vi "Test Asic DACTH0-5.vi"(0 "Config Test IN":T1={"Config HW"={"VISA Rigol DP832"="Rigol_DP832", "Config Rigol DP832"=[{"Channel"=0, "V Limit"=5.5, "I Limit"=0.5, "V Out"=5.0}, {"Channel"=1, "V Limit"=5.5, "I Limit"=0.8, "V Out"=5.0}, {"Channel"=2, "V Limit"=5.5, "I Limit"=0.2, "V Out"=0.0}], "CTA Test#"="CTA013 A", "FT_Handle"=0, "Espera acceso FT"=10}, "Config Test"=[{"Vasic"=3.3, "Test Register?"=TRUE, "Test ADC?"=TRUE, "Test ADC"={"Repeats ADC"=100, "Max Desviation"=0.1}, "Test Max PN Min NP?"=TRUE, "Pattern Max PN Min NP"={"Max P inferior"=1.888, "Max P superior"=2.177000045776367, "Min N superior"=0.818, "Min N inferior"=0.73, "Max N superior"=1.475, "Max N inferior"=1.322, "Min P inferior "=1.321, "Min P superior"=1.474}, "Test Rate Scan?"=TRUE, "Vin Rate Scan"=[0, 1, 2, 3, 4, 5, 6, 7, 8, 9], "Test Rate Scan Adders? 2"=TRUE, "Vin Rate Adders"=[0, 1], "Test offset analog?"=TRUE, "Test offset digital?"=TRUE}, {"Vasic"=3.2, "Test Register?"=TRUE, "Test ADC?"=TRUE, "Test ADC"={"Repeats ADC"=100, "Max Desviation"=0.1}, "Test Max PN Min NP?"=TRUE, "Pattern Max PN Min NP"={"Max P inferior"=1.888, "Max P superior"=2.177000045776367, "Min N superior"=0.818, "Min N inferior"=0.73, "Max N superior"=1.475, "Max N inferior"=1.322, "Min P inferior "=1.321, "Min P superior"=1.474}, "Test Rate Scan?"=TRUE, "Vin Rate Scan"=[0, 3], "Test Rate Scan Adders? 2"=TRUE, "Vin Rate Adders"=[0, 1], "Test offset analog?"=TRUE, "Test offset digital?"=TRUE}, {"Vasic"=3.1, "Test Register?"=TRUE, "Test ADC?"=TRUE, "Test ADC"={"Repeats ADC"=100, "Max Desviation"=0.1}, "Test Max PN Min NP?"=TRUE, "Pattern Max PN Min NP"={"Max P inferior"=1.888, "Max P superior"=2.177000045776367, "Min N superior"=0.818, "Min N inferior"=0.73, "Max N superior"=1.475, "Max N inferior"=1.322, "Min P inferior "=1.321, "Min P superior"=1.474}, "Test Rate Scan?"=TRUE, "Vin Rate Scan"=[0, 3], "Test Rate Scan Adders? 2"=TRUE, "Vin Rate Adders"=[0, 1], "Test offset analog?"=TRUE, "Test offset digital?"=TRUE}, {"Vasic"=3.0, "Test Register?"=TRUE, "Test ADC?"=TRUE, "Test ADC"={"Repeats ADC"=100, "Max Desviation"=0.1}, "Test Max PN Min NP?"=TRUE, "Pattern Max PN Min NP"={"Max P inferior"=1.888, "Max P superior"=2.177000045776367, "Min N superior"=0.818, "Min N inferior"=0.73, "Max N superior"=1.475, "Max N inferior"=1.322, "Min P inferior "=1.321, "Min P superior"=1.474}, "Test Rate Scan?"=TRUE, "Vin Rate Scan"=[0, 3], "Test Rate Scan Adders? 2"=TRUE, "Vin Rate Adders"=[0, 1], "Test offset analog?"=TRUE, "Test offset digital?"=TRUE}], "Result"=[], "Execucion Test"={"Vasic Actual"=0}} {"Config Test"."Pattern Max PN Min NP"."Min P superior" format="%.3g"; "Config Test"."Pattern Max PN Min NP"."Min P inferior" format="%.3g"; "Config Test"."Pattern Max PN Min NP"."Max N inferior" format="%.3g"; "Config Test"."Pattern Max PN Min NP"."Max N superior" format="%.3g"; "Config Test"."Pattern Max PN Min NP"."Min N inferior" format="%.3g"; "Config Test"."Pattern Max PN Min NP"."Min N superior" format="%.3g"; "Config Test"."Pattern Max PN Min NP"."Max P superior" format="%.3g"; "Config Test"."Pattern Max PN Min NP"."Max P inferior" format="%.3g"; "Config Test"."Vasic" min=2.8 max=3.8 step=0.01 format="%.2g"; "Config HW"."Config Rigol DP832"."Channel" items=["+30V Channel 1", "+30V Channel 2", "+5V Channel 3"]; "Config HW"."Config Rigol DP832"."V Limit" format="%.1g"; "Config HW"."Config Rigol DP832"."I Limit" format="%.1g"; "Config HW"."Config Rigol DP832"."V Out" format="%.1g"; "Result"."Test Registros"."Read W/R" format="%04x"; "Result"."Test Registros"."Pattern W/R" format="%04x"; "Result"."Test Registros"."Read Default" format="%04x"; "Result"."Test Registros"."Pattern Default" format="%04x"}, 11 "Error IN":errorcluster) -> (4 "Config Test OUT":T1={"Config HW"={"VISA Rigol DP832"="Rigol_DP832", "Config Rigol DP832"=[{"Channel"=0, "V Limit"=5.5, "I Limit"=0.5, "V Out"=5.0}, {"Channel"=1, "V Limit"=5.5, "I Limit"=0.8, "V Out"=5.0}, {"Channel"=2, "V Limit"=5.5, "I Limit"=0.2, "V Out"=0.0}], "CTA Test#"="CTA013 A", "FT_Handle"=0, "Espera acceso FT"=10}, "Config Test"=[{"Vasic"=3.3, "Test Register?"=TRUE, "Test ADC?"=TRUE, "Test ADC"={"Repeats ADC"=100, "Max Desviation"=0.1}, "Test Max PN Min NP?"=TRUE, "Pattern Max PN Min NP"={"Max P inferior"=1.888, "Max P superior"=2.177000045776367, "Min N superior"=0.818, "Min N inferior"=0.73, "Max N superior"=1.475, "Max N inferior"=1.322, "Min P inferior "=1.321, "Min P superior"=1.474}, "Test Rate Scan?"=TRUE, "Vin Rate Scan"=[0, 1, 2, 3, 4, 5, 6, 7, 8, 9], "Test Rate Scan Adders? 2"=TRUE, "Vin Rate Adders"=[0, 1], "Test offset analog?"=TRUE, "Test offset digital?"=TRUE}, {"Vasic"=3.2, "Test Register?"=TRUE, "Test ADC?"=TRUE, "Test ADC"={"Repeats ADC"=100, "Max Desviation"=0.1}, "Test Max PN Min NP?"=TRUE, "Pattern Max PN Min NP"={"Max P inferior"=1.888, "Max P superior"=2.177000045776367, "Min N superior"=0.818, "Min N inferior"=0.73, "Max N superior"=1.475, "Max N inferior"=1.322, "Min P inferior "=1.321, "Min P superior"=1.474}, "Test Rate Scan?"=TRUE, "Vin Rate Scan"=[0, 3], "Test Rate Scan Adders? 2"=TRUE, "Vin Rate Adders"=[0, 1], "Test offset analog?"=TRUE, "Test offset digital?"=TRUE}, {"Vasic"=3.1, "Test Register?"=TRUE, "Test ADC?"=TRUE, "Test ADC"={"Repeats ADC"=100, "Max Desviation"=0.1}, "Test Max PN Min NP?"=TRUE, "Pattern Max PN Min NP"={"Max P inferior"=1.888, "Max P superior"=2.177000045776367, "Min N superior"=0.818, "Min N inferior"=0.73, "Max N superior"=1.475, "Max N inferior"=1.322, "Min P inferior "=1.321, "Min P superior"=1.474}, "Test Rate Scan?"=TRUE, "Vin Rate Scan"=[0, 3], "Test Rate Scan Adders? 2"=TRUE, "Vin Rate Adders"=[0, 1], "Test offset analog?"=TRUE, "Test offset digital?"=TRUE}, {"Vasic"=3.0, "Test Register?"=TRUE, "Test ADC?"=TRUE, "Test ADC"={"Repeats ADC"=100, "Max Desviation"=0.1}, "Test Max PN Min NP?"=TRUE, "Pattern Max PN Min NP"={"Max P inferior"=1.888, "Max P superior"=2.177000045776367, "Min N superior"=0.818, "Min N inferior"=0.73, "Max N superior"=1.475, "Max N inferior"=1.322, "Min P inferior "=1.321, "Min P superior"=1.474}, "Test Rate Scan?"=TRUE, "Vin Rate Scan"=[0, 3], "Test Rate Scan Adders? 2"=TRUE, "Vin Rate Adders"=[0, 1], "Test offset analog?"=TRUE, "Test offset digital?"=TRUE}], "Result"=[], "Execucion Test"={"Vasic Actual"=0}} {"Config Test"."Pattern Max PN Min NP"."Min P superior" format="%.3g"; "Config Test"."Pattern Max PN Min NP"."Min P inferior" format="%.3g"; "Config Test"."Pattern Max PN Min NP"."Max N inferior" format="%.3g"; "Config Test"."Pattern Max PN Min NP"."Max N superior" format="%.3g"; "Config Test"."Pattern Max PN Min NP"."Min N inferior" format="%.3g"; "Config Test"."Pattern Max PN Min NP"."Min N superior" format="%.3g"; "Config Test"."Pattern Max PN Min NP"."Max P superior" format="%.3g"; "Config Test"."Pattern Max PN Min NP"."Max P inferior" format="%.3g"; "Config Test"."Vasic" min=2.8 max=3.8 step=0.01 format="%.2g"; "Config HW"."Config Rigol DP832"."Channel" items=["+30V Channel 1", "+30V Channel 2", "+5V Channel 3"]; "Config HW"."Config Rigol DP832"."V Limit" format="%.1g"; "Config HW"."Config Rigol DP832"."I Limit" format="%.1g"; "Config HW"."Config Rigol DP832"."V Out" format="%.1g"; "Result"."Test Registros"."Read W/R" format="%04x"; "Result"."Test Registros"."Pattern W/R" format="%04x"; "Result"."Test Registros"."Read Default" format="%04x"; "Result"."Test Registros"."Pattern Default" format="%04x"}, 8 "Max P Min N":bool, 10 "Min P Max N":bool, 15 "Error OUT":errorcluster)   [LabVIEW 2009]
uses:
  Test.ctl
  Test_config.ctl
  Rigol DP832/DP832_Control Channels.ctl
  Valores configuracion test.ctl
  Test_result.ctl
  test_result fvasic.ctl
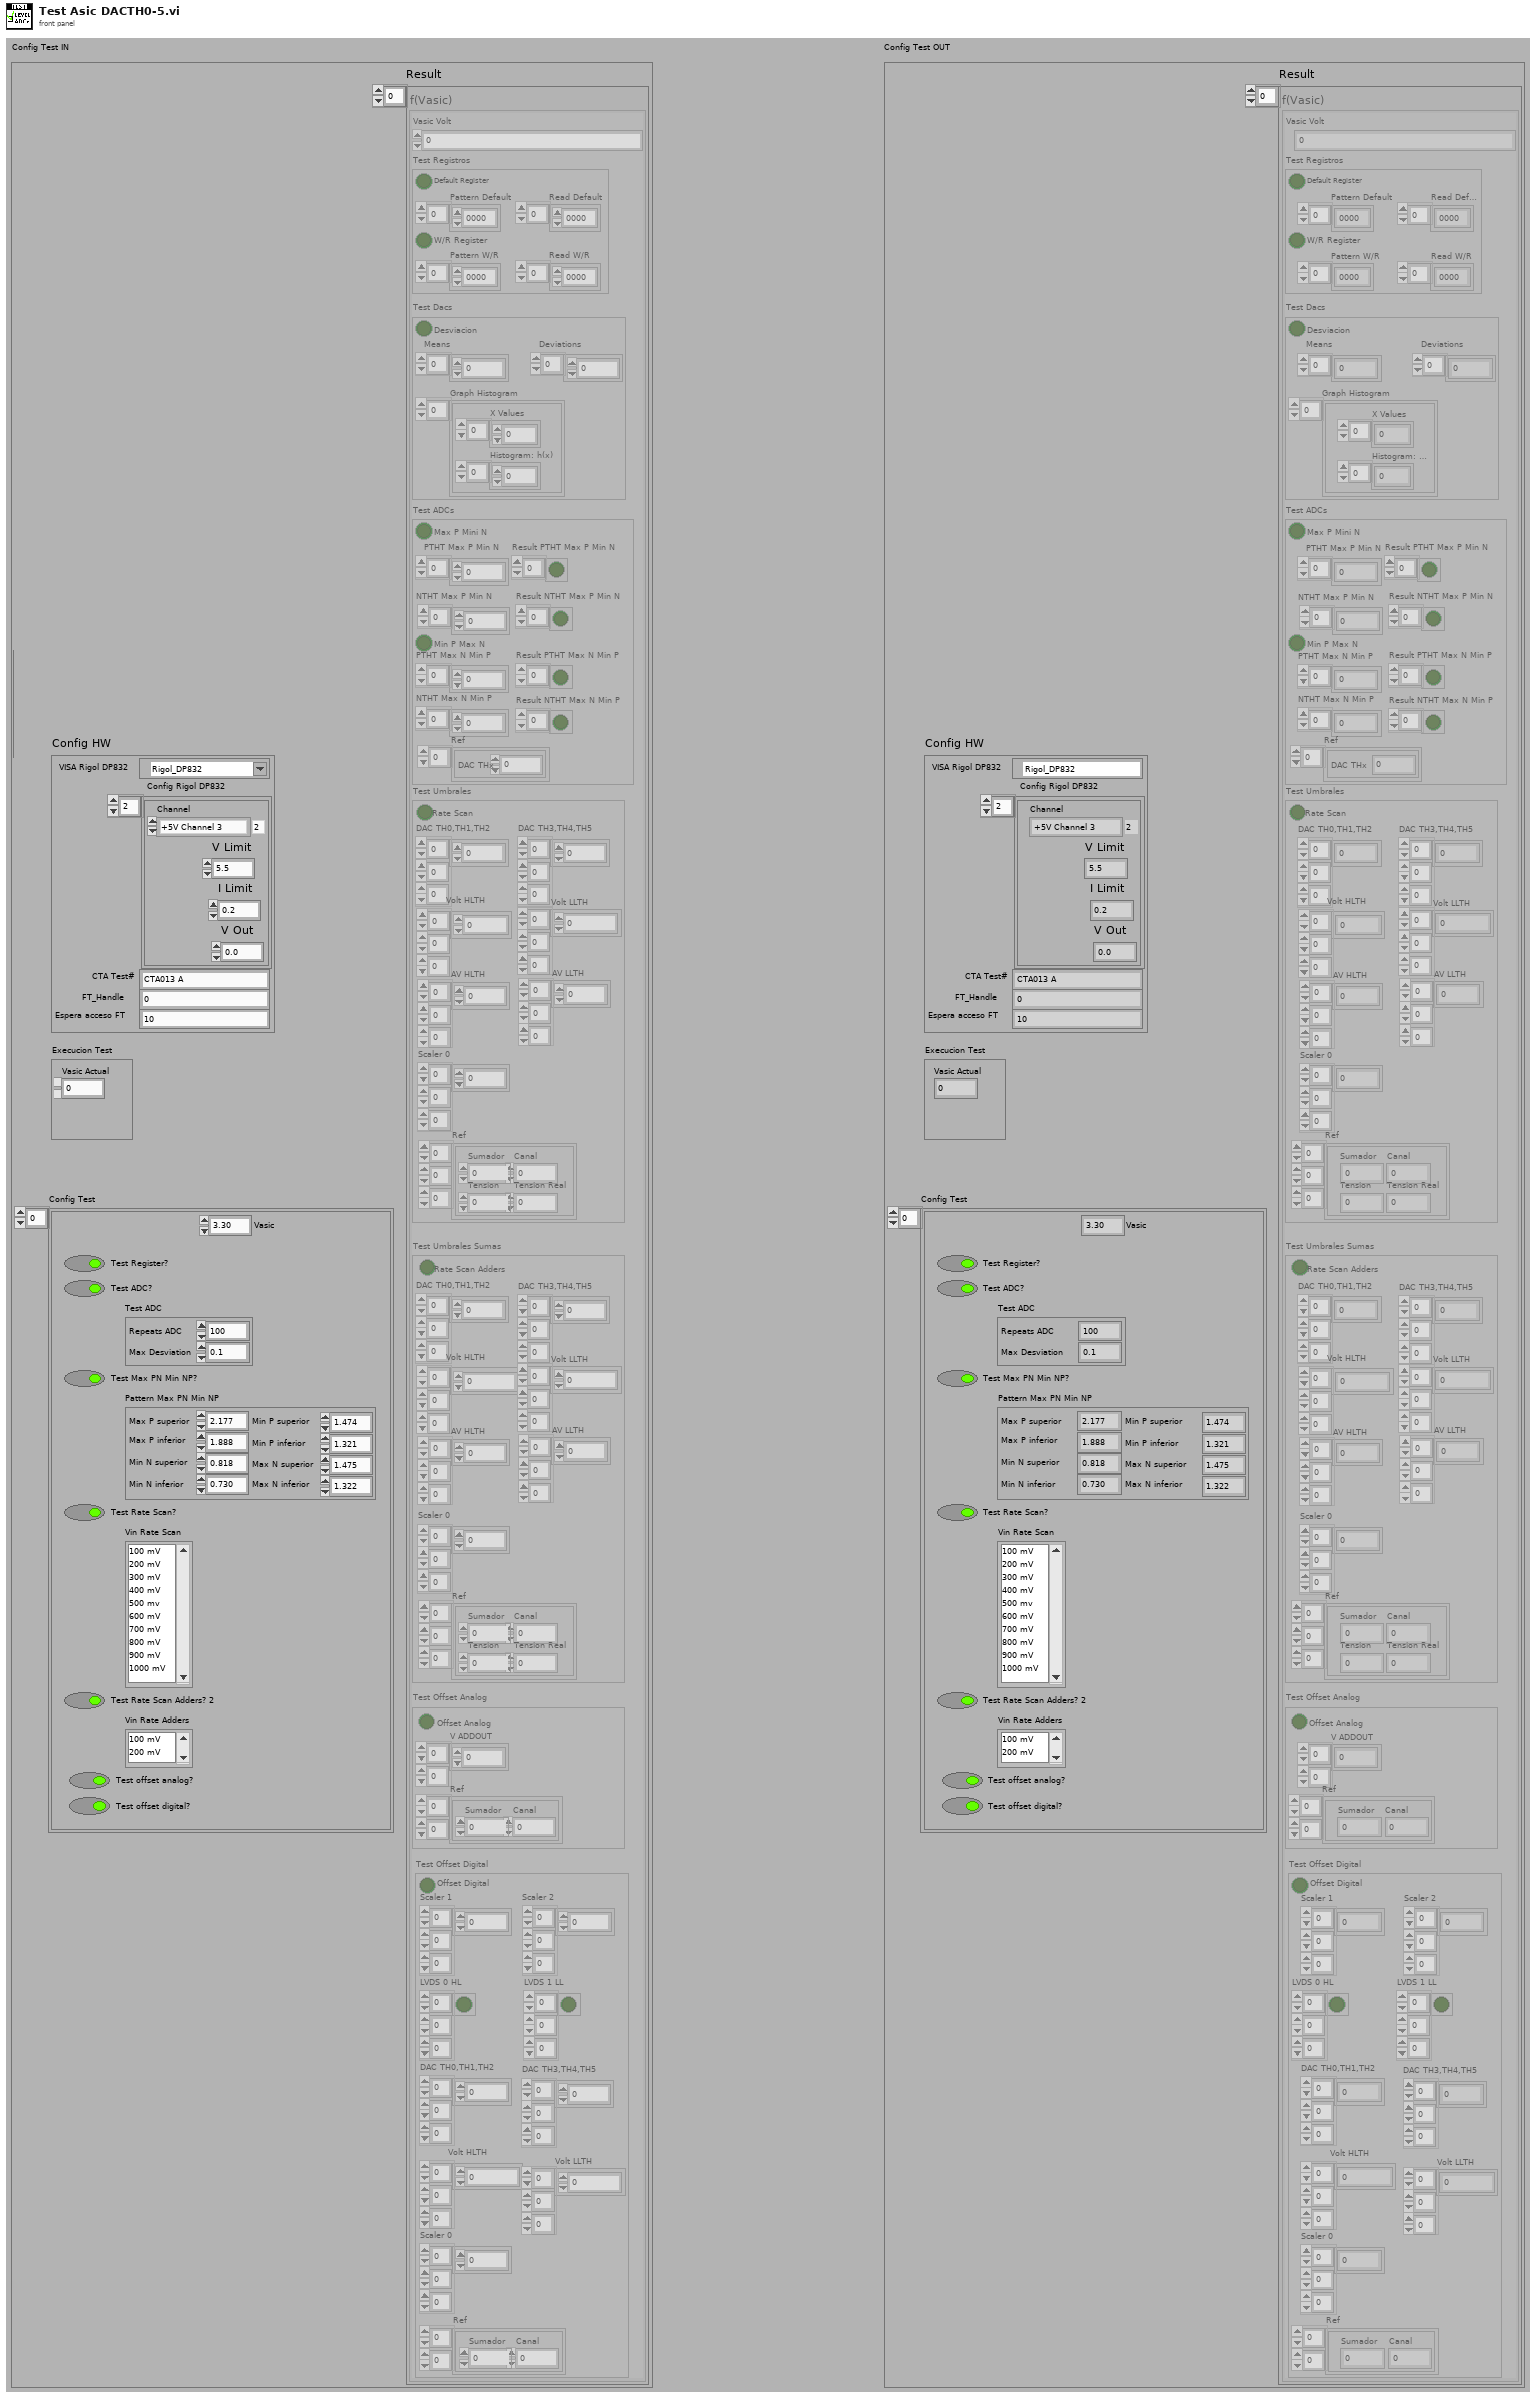
[diagram p1: front panel]
types:
  T1 = typedef "Test.ctl" = cluster{"Config HW":T2, "Config Test":T4, "Result":T5, "Execucion Test":cluster{"Vasic Actual":i32}}
  T2 = typedef "Test_config.ctl" = cluster{"VISA Rigol DP832":refnum<visa-resource-name>, "Config Rigol DP832":cluster{"Channel":T3, "V Limit":dbl, "I Limit":dbl, "V Out":dbl}[], "CTA Test#":string, "FT_Handle":u32, "Espera acceso FT":u32}
  T3 = typedef "DP832_Control Channels.ctl" = i32
  T4 = typedef "Valores configuracion test.ctl" = cluster{"Vasic":dbl, "Test Register?":bool, "Test ADC?":bool, "Test ADC":cluster{"Repeats ADC":i32, "Max Desviation":dbl}, "Test Max PN Min NP?":bool, "Pattern Max PN Min NP":cluster{"Max P inferior":dbl, "Max P superior":dbl, "Min N superior":dbl, "Min N inferior":dbl, "Max N superior":dbl, "Max N inferior":dbl, "Min P inferior ":dbl, "Min P superior":dbl}, "Test Rate Scan?":bool, "Vin Rate Scan":i32[], "Test Rate Scan Adders? 2":bool, "Vin Rate Adders":i32[], "Test offset analog?":bool, "Test offset digital?":bool}[]
  T5 = typedef "Test_result.ctl" = T6[]
  T6 = typedef "test_result fvasic.ctl" = cluster{"Vasic Volt":i32, "Test Registros":cluster{"Default Register":bool, "Pattern Default":u16[], "Read Default":u16[], "W/R Register":bool, "Pattern W/R":u16[], "Read W/R":u16[]}, "Test Dacs":cluster{"Desviacion":bool, "Means":dbl[], "Deviations":dbl[], "Graph Histogram":cluster{"X Values":dbl[], "Histogram: h(x)":i32[]}[]}, "Test ADCs":cluster{"Max P Mini N":bool, "PTHT Max P Min N":dbl[], "Result PTHT Max P Min N":bool[], "NTHT Max P Min N":dbl[], "Result NTHT Max P Min N":bool[], "Min P Max N":bool, "PTHT Max N Min P":dbl[], "Result PTHT Max N Min P":bool[], "NTHT Max N Min P":dbl[], "Result NTHT Max N Min P":bool[], "Ref":cluster{"DAC THx":u8}[]}, "Test Umbrales":cluster{"Rate Scan":bool, "DAC TH0,TH1,TH2":u16[][][], "Volt HLTH":dbl[][][], "AV HLTH":dbl[][][], "DAC TH3,TH4,TH5":u16[][][], "Volt LLTH":dbl[][][], "AV LLTH":dbl[][][], "Scaler 0":u16[][][], "Ref":cluster{"Sumador":u8, "Canal":u8, "Tension":u8, "Tension Real":dbl}[][][]}, "Test Umbrales Sumas":cluster{"Rate Scan Adders":bool, "DAC TH0,TH1,TH2":u16[][][], "Volt HLTH":dbl[][][], "AV HLTH":dbl[][][], "DAC TH3,TH4,TH5":u16[][][], "Volt LLTH":dbl[][][], "AV LLTH":dbl[][][], "Scaler 0":u16[][][], "Ref":cluster{"Sumador":u8, "Canal":u8, "Tension":u8, "Tension Real":dbl}[][][]}, "Test Offset Analog":cluster{"Offset Analog":bool, "V ADDOUT":dbl[][], "Ref":cluster{"Sumador":u8, "Canal":u8}[][]}, "Test Offset Digital":cluster{"Offset Digital":bool, "Scaler 1":u16[][][], "LVDS 0 HL":bool[][][], "DAC TH0,TH1,TH2":u16[][][], "Volt HLTH":dbl[][][], "Scaler 2":u16[][][], "LVDS 1 LL":bool[][][], "DAC TH3,TH4,TH5":u16[][][], "Volt LLTH":dbl[][][], "Scaler 0":u16[][][], "Ref":cluster{"Sumador":u8, "Canal":u8}[][]}}
  T7 = cluster{"Vasic":dbl, "Test Register?":bool, "Test ADC?":bool, "Test ADC":cluster{"Repeats ADC":i32, "Max Desviation":dbl}, "Test Max PN Min NP?":bool, "Pattern Max PN Min NP":cluster{"Max P inferior":dbl, "Max P superior":dbl, "Min N superior":dbl, "Min N inferior":dbl, "Max N superior":dbl, "Max N inferior":dbl, "Min P inferior ":dbl, "Min P superior":dbl}, "Test Rate Scan?":bool, "Vin Rate Scan":i32[], "Test Rate Scan Adders? 2":bool, "Vin Rate Adders":i32[], "Test offset analog?":bool, "Test offset digital?":bool}
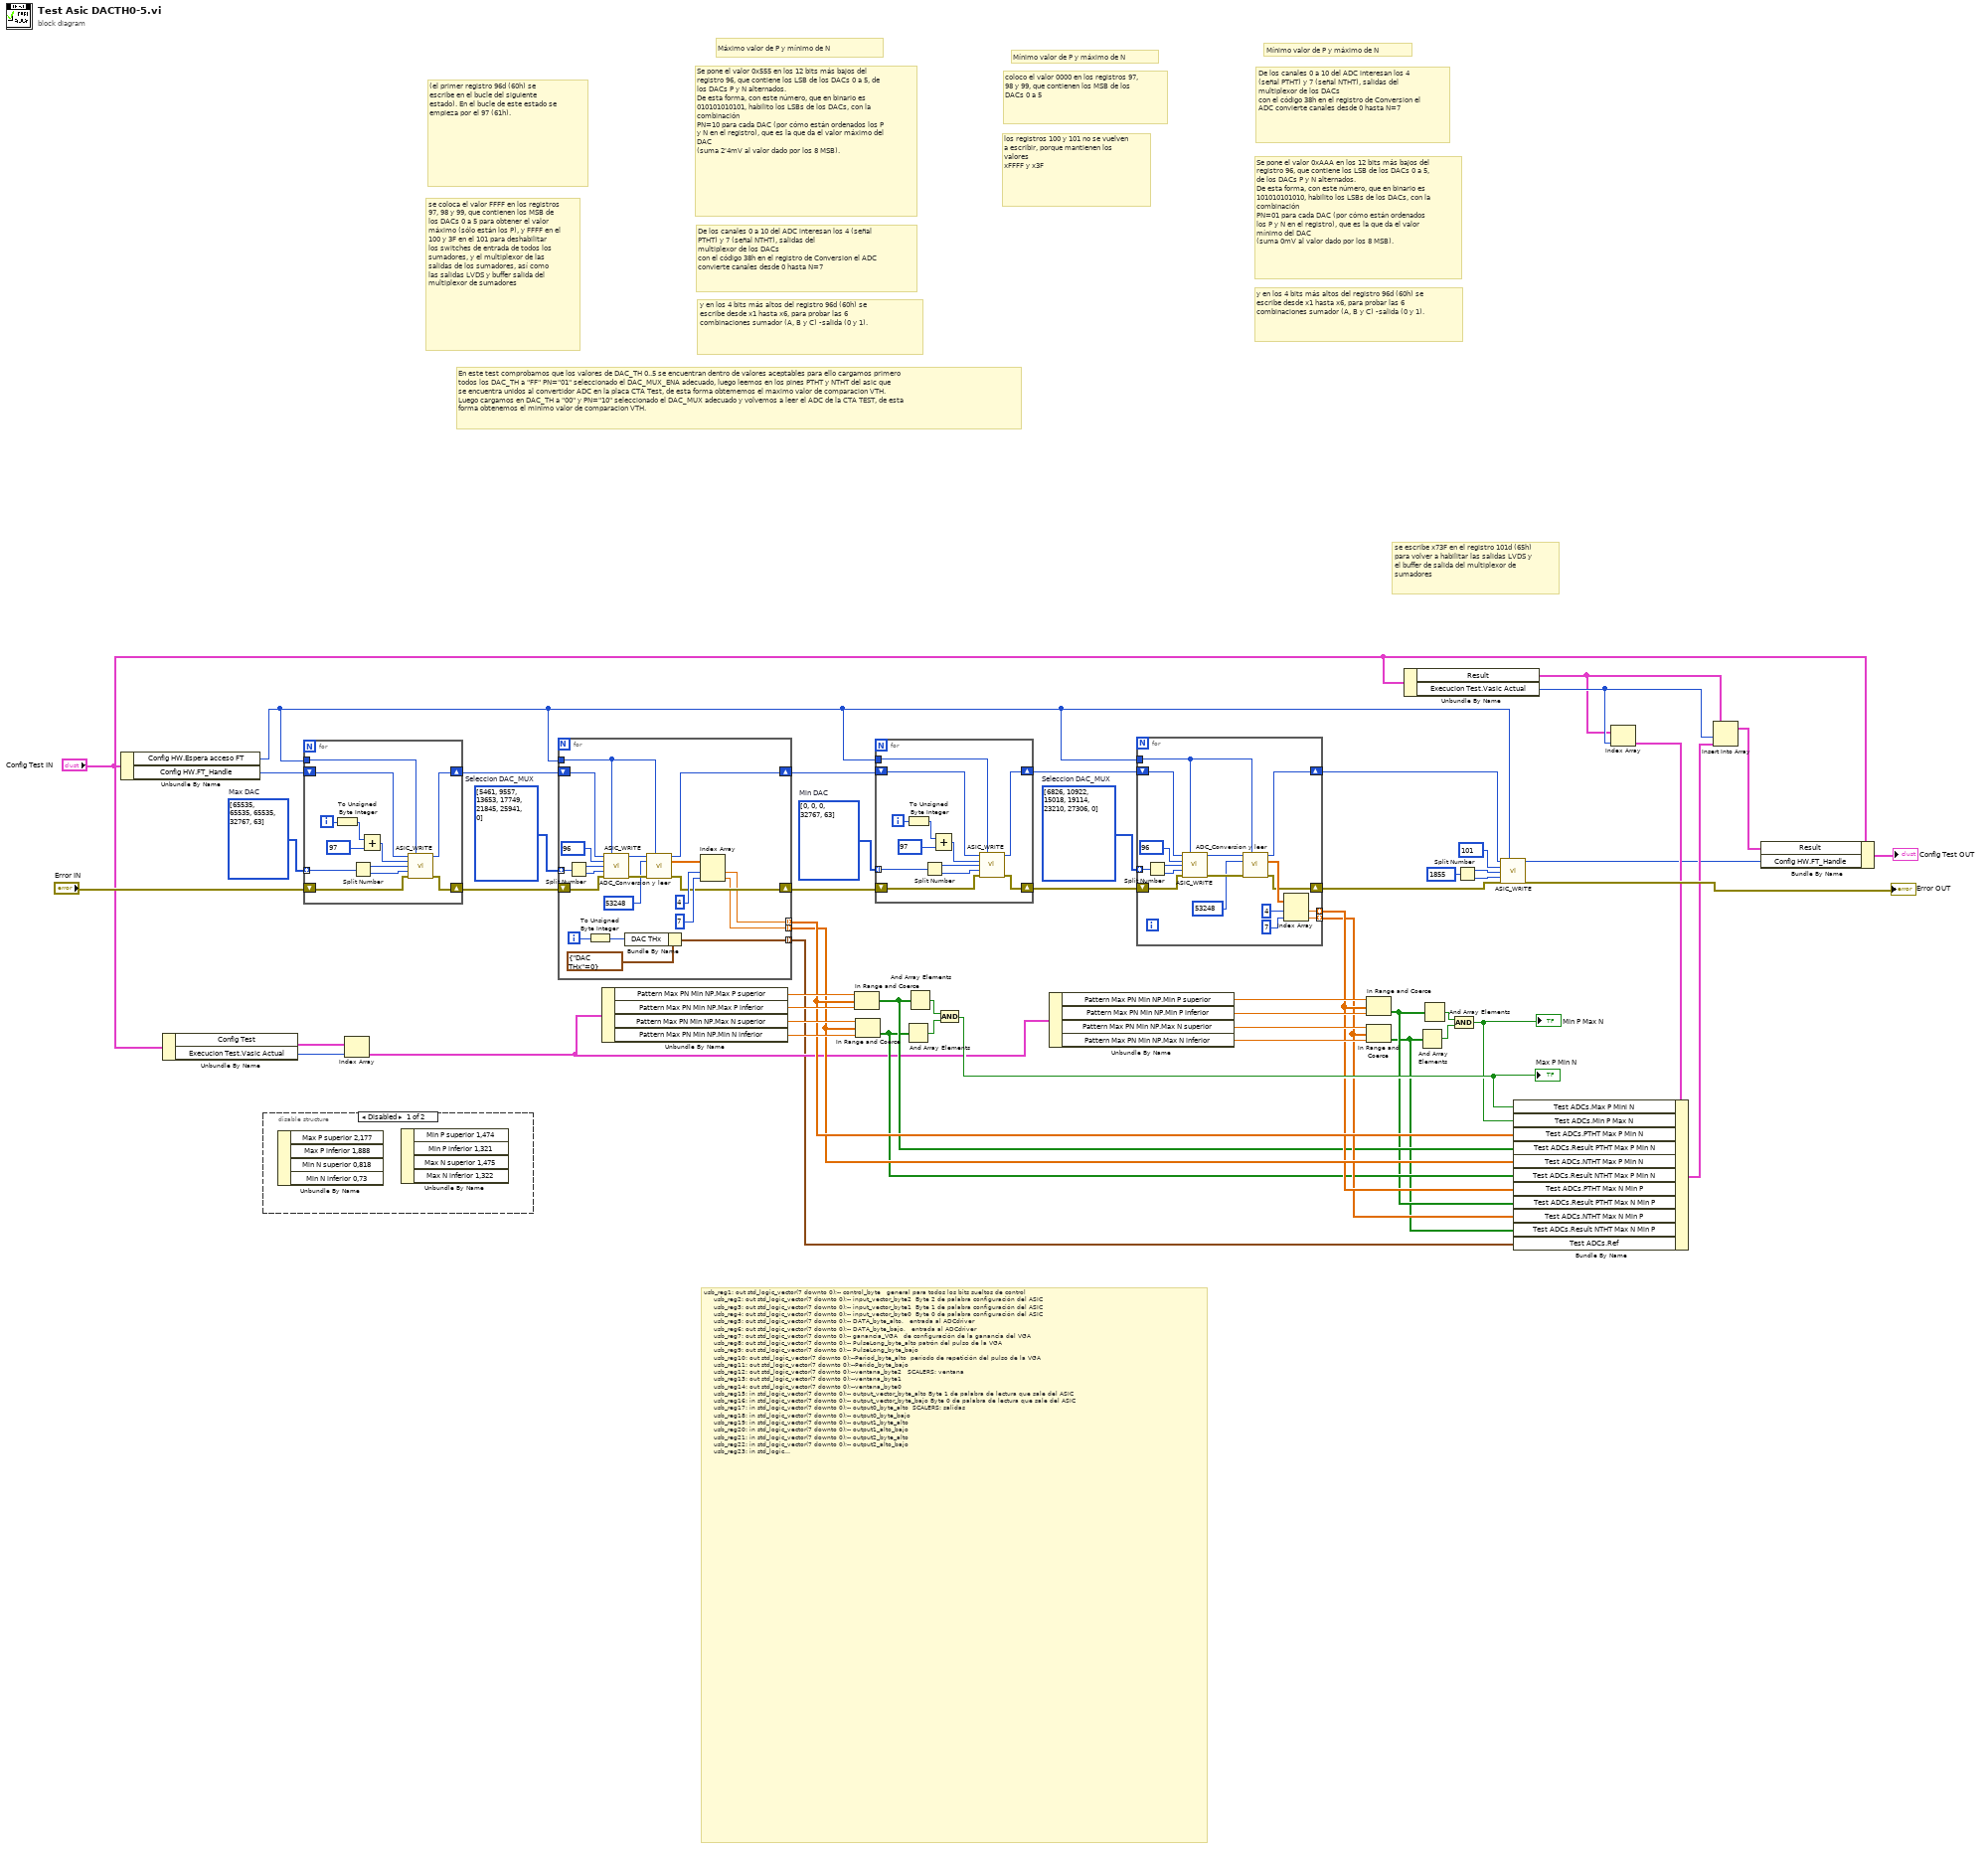
[diagram p0: block diagram]
diagram:
  w43 = u16[] [6826, 10922, 15018, 19114, 23210, 27306, 0]  # Seleccion DAC_MUX
  w45 = u16[] [0, 0, 0, 32767, 63]  # Min DAC
  w50 = u16[] [5461, 9557, 13653, 17749, 21845, 25941, 0]  # Seleccion DAC_MUX
  w52 = u16[] [65535, 65535, 65535, 32767, 63]  # Max DAC
  # "En este test comprobamos que los valores de DAC_TH 0..5 se encuentran dentro de valores aceptables para ello cargamos primero\ntodos los DAC_TH a \"FF\" PN=\"01\" seleccionado el DAC_MUX_ENA adecuado, luego leemos en los pines PTHT y NTHT del asic que \nse encuentra unidos al convertidor ADC en la placa CTA Test, de esta forma obtememos el maximo valor de comparacion VTH.\nLuego cargamos en DAC_TH a \"00\" y PN=\"10\" seleccionado el DAC_MUX adecuado y volvemos a leer el ADC de la CTA TEST, de esta\nforma obtenemos el minimo valor de comparacion VTH."
  # "se escribe x73F en el registro 101d (65h) para volver a habilitar las salidas LVDS y el buffer de salida del multiplexor de sumadores"
  # "Mínimo valor de P y máximo de N"
  # "De los canales 0 a 10 del ADC interesan los 4 (señal PTHT) y 7 (señal NTHT), salidas del\nmultiplexor de los DACs\ncon el código 38h en el registro de Conversion el ADC convierte canales desde 0 hasta N=7"
  # "Se pone el valor 0xAAA en los 12 bits más bajos del registro 96, que contiene los LSB de los DACs 0 a 5, de los DACs P y N alternados.\nDe esta forma, con este número, que en binario es 101010101010, habilito los LSBs de los DACs, con la combinación\nPN=01 para cada DAC (por cómo están ordenados los P y N en el registro), que es la que da el valor mínimo del DAC \n(suma 0mV al valor dado por los 8 MSB)."
  # "y en los 4 bits más altos del registro 96d (60h) se escribe desde x1 hasta x6, para probar las 6 combinaciones sumador (A, B y C) -salida (0 y 1)."
  # "los registros 100 y 101 no se vuelven \na escribir, porque mantienen los valores \nxFFFF y x3F"
  # "coloco el valor 0000 en los registros 97, 98 y 99, que contienen los MSB de los DACs 0 a 5"
  # "Mínimo valor de P y máximo de N"
  # "y en los 4 bits más altos del registro 96d (60h) se escribe desde x1 hasta x6, para probar las 6 combinaciones sumador (A, B y C) -salida (0 y 1)."
  # "Se pone el valor 0x555 en los 12 bits más bajos del registro 96, que contiene los LSB de los DACs 0 a 5, de los DACs P y N alternados.\nDe esta forma, con este número, que en binario es 010101010101, habilito los LSBs de los DACs, con la combinación\nPN=10 para cada DAC (por cómo están ordenados los P y N en el registro), que es la que da el valor máximo del DAC \n(suma 2'4mV al valor dado por los 8 MSB)."
  # "Máximo valor de P y mínimo de N"
  # "De los canales 0 a 10 del ADC interesan los 4 (señal PTHT) y 7 (señal NTHT), salidas del\nmultiplexor de los DACs\ncon el código 38h en el registro de Conversion el ADC convierte canales desde 0 hasta N=7"
  # "(el primer registro 96d (60h) se\nescribe en el bucle del siguiente \nestado). En el bucle de este estado se empieza por el 97 (61h)."
  # "se coloca el valor FFFF en los registros 97, 98 y 99, que contienen los MSB de los DACs 0 a 5 para obtener el valor máximo (sólo están los P), y FFFF en el 100 y 3F en el 101 para deshabilitar los switches de entrada de todos los sumadores, y el multiplexor de las salidas de los sumadores, así como las salidas LVDS y buffer salida del multiplexor de sumadores"
  # "usb_reg1: out std_logic_vector(7 downto 0);-- control_byte\t\t\tgeneral para todos los bits sueltos de control\n\t\t\t  usb_reg2: out std_logic_vector(7 downto 0);-- input_vector_byte2 \tByte 2 de palabra configuración del ASIC\n\t\t\t  usb_reg3: out std_logic_vector(7 downto 0);-- input_vector_byte1 \tByte 1 de palabra configuración del ASIC\n\t\t\t  usb_reg4: out std_logic_vector(7 downto 0);-- input_vector_byte0 \tByte 0 de palabra configuración del ASIC\n\t\t\t  usb_reg5: out std_logic_vector(7 downto 0);-- DATA_byte_alto, \t\tentrada al ADCdriver\n\t\t\t  usb_reg6: out std_logic_vector(7 downto 0);-- DATA_byte_bajo, \t\tentrada al ADCdriver\n\t\t\t  usb_reg7: out std_logic_vector(7 downto 0);-- ganancia_VGA\t\t\tde configuración de la ganancia del VGA\n\t\t\t  usb_reg8: out std_logic_vector(7 downto 0);-- PulseLong_byte_alto\tpatrón del pulso de la VGA\n\t\t\t  usb_reg9: out std_logic_vector(7 downto 0);-- PulseLong_byte_bajo\n\t\t\t  usb_reg10: out std_logic_vector(7 downto 0);--Period_byte_alto\t\tperíodo de repetición del pulso de la VGA\n\t\t\t  usb_reg11: out std_logic_vector(7 downto 0);--Perido_byte_bajo\n\t\t\t  usb_reg12: out std_logic_vector(7 downto 0);--ventana_byte2\t\t\tSCALERS: ventana\n\t\t\t  usb_reg13: out std_logic_vector(7 downto 0);--ventana_byte1\t\n\t\t\t  usb_reg14: out std_logic_vector(7 downto 0);--ventana_byte0\n\t\t\t  usb_reg15: in std_logic_vector(7 downto 0);-- output_vector_byte_alto\tByte 1 de palabra de lectura que sale del ASIC\n\t\t\t  usb_reg16: in std_logic_vector(7 downto 0);-- output_vector_byte_bajo\tByte 0 de palabra de lectura que sale del ASIC\n\t\t\t  usb_reg17: in std_logic_vector(7 downto 0);-- output0_byte_alto\t\tSCALERS: salidas\n\t\t\t  usb_reg18: in std_logic_vector(7 downto 0);-- output0_byte_bajo\n\t\t\t  usb_reg19: in std_logic_vector(7 downto 0);-- output1_byte_alto\n\t\t\t  usb_reg20: in std_logic_vector(7 downto 0);-- output1_alto_bajo \n\t\t\t  usb_reg21: in std_logic_vector(7 downto 0);-- output2_byte_alto \n\t\t\t  usb_reg22: in std_logic_vector(7 downto 0);-- output2_alto_bajo \n\t\t\t  usb_reg23: in std_logic_vector(7 downto 0);-- para el canal_0 del ADCdriver\n\t\t\t  usb_reg24: in std_logic_vector(7 downto 0);\n\t\t\t  usb_reg25: in std_logic_vector(7 downto 0);-- para el canal_1 del ADCdriver\n\t\t\t  usb_reg26: in std_logic_vector(7 downto 0);\n\t\t\t  usb_reg27: in std_logic_vector(7 downto 0);-- para el canal_2 del ADCdriver\n\t\t\t  usb_reg28: in std_logic_vector(7 downto 0);\n\t\t\t  usb_reg29: in std_logic_vector(7 downto 0);-- para el canal_3 del ADCdriver\n\t\t\t  usb_reg30: in std_logic_vector(7 downto 0);\n\t\t\t  usb_reg31: in std_logic_vector(7 downto 0);-- para el canal_4 del ADCdriver\n\t\t\t  usb_reg32: in std_logic_vector(7 downto 0);\n\t\t\t  usb_reg33: in std_logic_vector(7 downto 0);-- para el canal_5 del ADCdriver\n\t\t\t  usb_reg34: in std_logic_vector(7 downto 0);\n\t\t\t  usb_reg35: in std_logic_vector(7 downto 0);-- para el canal_6 del ADCdriver\n\t\t\t  usb_reg36: in std_logic_vector(7 downto 0);\n\t\t\t  usb_reg37: in std_logic_vector(7 downto 0);-- para el canal_7 del ADCdriver\n\t\t\t  usb_reg38: in std_logic_vector(7 downto 0);\n\t\t\t  usb_reg39: in std_logic_vector(7 downto 0);-- para el canal_8 del ADCdriver\n\t\t\t  usb_reg40: in std_logic_vector(7 downto 0);\n\t\t\t  usb_reg41: in std_logic_vector(7 downto 0);-- para el canal_9 del ADCdriver\n\t\t\t  usb_reg42: in std_logic_vector(7 downto 0);\n\t\t\t  usb_reg43: in std_logic_vector(7 downto 0);-- para el canal_10 del ADCdriver\n\t\t\t  usb_reg44: in std_logic_vector(7 downto 0)--;  \n\n     usb_reg55 => LVDSByte"
  n1 = Unbundle By Name("Config Test IN") -> ("Config HW.Espera acceso FT"=w35:u32, "Config HW.FT_Handle"=w51:u32)
  n2 = Unbundle By Name("Config Test IN") -> ("Config Test"=w4:T4, "Execucion Test.Vasic Actual"=w3:i32)
  n3 = disable-structure shown="Disabled" {
    frame #0 {
      n4 = Unbundle By Name() -> ()  [unwired: 1 in, 4 out]
      n5 = Unbundle By Name() -> ()  [unwired: 1 in, 4 out]
    }
    frame #1 {
    }
  }
  n6 = for {
    tunnel: w52 -> [w64] mode=indexing
    shift-right: [w62] -> w49
    shift-left: "Error IN" -> [w63]
    tunnel: w35 -> [w58]
    shift-right: [w55] -> w48
    shift-left: w51 -> [w56]
    i -> [w61]
    n7 = To Unsigned Byte Integer(number=w61) -> (unsigned 8bit integer=w60:u8)
    n8 = Split Number(x=w64) -> (hi(x)=w65:u8, lo(x)=w66:u8)
    n9 = Add(x=w60, y=u8 97 ("devNum_in")) -> (x+y=w57:u8)
    n10 = call "ASIC_WRITE.vi"("ftHandle_in"=w56, "Espera acceso USB"=w58, "Direccion Registro Asic"=w57, "Byte Alto"=w65, "Byte Bajo"=w66, "error in"=w63) -> ("ftHandle_out"=w55:u32, "error out"=w62:errorcluster)  [unwired: 8 in]
  }
  n11 = Index Array(array=w4, index=w3) -> (element=w7:T7)
  n12 = for {
    tunnel: w50 -> [w85] mode=indexing
    shift-right: [w75] -> w47
    shift-left: w49 -> [w84]
    tunnel: w35 -> [w80]
    shift-right: [w76] -> w46
    shift-left: w48 -> [w83]
    tunnel: [w73] -> w15 mode=indexing
    tunnel: [w72] -> w14 mode=indexing
    tunnel: [w67] -> w1 mode=indexing
    i -> [w71]
    n13 = Split Number(x=w85) -> (hi(x)=w86:u8, lo(x)=w87:u8)
    n14 = To Unsigned Byte Integer(number=w71) -> (unsigned 8bit integer=w69:u8)
    n15 = call "ASIC_WRITE.vi"("ftHandle_in"=w83, "Espera acceso USB"=w80, "Direccion Registro Asic"=u8 96 ("devNum_in"), "Byte Alto"=w86, "Byte Bajo"=w87, "error in"=w84) -> ("ftHandle_out"=w81:u32, "error out"=w82:errorcluster)  [unwired: 8 in]
    n16 = Bundle By Name(cluster=cluster{"DAC THx":u8} {"DAC THx"=0}, "DAC THx"=w69) -> (w67:cluster{"DAC THx":u8})
    n17 = call "ADC_Conversion y leer.vi"("ftHandle_in 2"=w81, "Espera acceso USB"=w80, "Registro Conversion (0xD000)"=u16 53248, "error in 2"=w82) -> ("ftHandle_out"=w76:u32, "Datos Canal (V)"=w79:dbl[], "error out"=w75:errorcluster)  [unwired: 6 in, 3 out]
    n18 = Index Array(array=w79, index #1=4 ("index"), index #2=7 ("index")) -> (element #1=w73:dbl, element #2=w72:dbl)
  }
  n19 = Unbundle By Name(w7) -> ("Pattern Max PN Min NP.Max P superior"=w29:dbl, "Pattern Max PN Min NP.Max P inferior"=w28:dbl, "Pattern Max PN Min NP.Max N superior"=w27:dbl, "Pattern Max PN Min NP.Min N inferior"=w26:dbl)
  n20 = In Range and Coerce(upper limit=w29, x=w15, lower limit=w28) -> (In Range?=w11:bool[])  [unwired: 1 out]
  n21 = In Range and Coerce(upper limit=w27, x=w14, lower limit=w26) -> (In Range?=w10:bool[])  [unwired: 1 out]
  n22 = for {
    tunnel: w45 -> [w97] mode=indexing
    shift-right: [w95] -> w42
    shift-left: w47 -> [w96]
    tunnel: w35 -> [w91]
    shift-right: [w88] -> w44
    shift-left: w46 -> [w89]
    i -> [w94]
    n23 = To Unsigned Byte Integer(number=w94) -> (unsigned 8bit integer=w93:u8)
    n24 = Split Number(x=w97) -> (hi(x)=w98:u8, lo(x)=w99:u8)
    n25 = Add(x=w93, y=u8 97 ("devNum_in")) -> (x+y=w90:u8)
    n26 = call "ASIC_WRITE.vi"("ftHandle_in"=w89, "Espera acceso USB"=w91, "Direccion Registro Asic"=w90, "Byte Alto"=w98, "Byte Bajo"=w99, "error in"=w96) -> ("ftHandle_out"=w88:u32, "error out"=w95:errorcluster)  [unwired: 8 in]
  }
  n27 = And Array Elements(Boolean array=w10) -> (logical AND=w25:bool)
  n28 = And Array Elements(Boolean array=w11) -> (logical AND=w24:bool)
  n29 = And(x=w24, y=w25) -> (x .and. y?=w23:bool)
  "Max P Min N" <- w23
  n30 = Unbundle By Name(w7) -> ("Pattern Max PN Min NP.Min P superior"=w22:dbl, "Pattern Max PN Min NP.Min P inferior"=w21:dbl, "Pattern Max PN Min NP.Max N superior"=w20:dbl, "Pattern Max PN Min NP.Max N inferior"=w19:dbl)
  n31 = for {
    tunnel: w43 -> [w114] mode=indexing
    shift-right: [w103] -> w36
    shift-left: w42 -> [w113]
    tunnel: w35 -> [w109]
    shift-right: [w104] -> w37
    shift-left: w44 -> [w112]
    tunnel: [w101] -> w13 mode=indexing
    tunnel: [w100] -> w12 mode=indexing
    n32 = Split Number(x=w114) -> (hi(x)=w115:u8, lo(x)=w116:u8)
    n33 = call "ASIC_WRITE.vi"("ftHandle_in"=w112, "Espera acceso USB"=w109, "Direccion Registro Asic"=u8 96 ("devNum_in"), "Byte Alto"=w115, "Byte Bajo"=w116, "error in"=w113) -> ("ftHandle_out"=w110:u32, "error out"=w111:errorcluster)  [unwired: 8 in]
    n34 = call "ADC_Conversion y leer.vi"("ftHandle_in 2"=w110, "Espera acceso USB"=w109, "Registro Conversion (0xD000)"=u16 53248, "error in 2"=w111) -> ("ftHandle_out"=w104:u32, "Datos Canal (V)"=w107:dbl[], "error out"=w103:errorcluster)  [unwired: 6 in, 3 out]
    n35 = Index Array(array=w107, index #1=4 ("index"), index #2=7 ("index")) -> (element #1=w101:dbl, element #2=w100:dbl)
  }
  n36 = In Range and Coerce(upper limit=w22, x=w13, lower limit=w21) -> (In Range?=w9:bool[])  [unwired: 1 out]
  n37 = In Range and Coerce(upper limit=w20, x=w12, lower limit=w19) -> (In Range?=w8:bool[])  [unwired: 1 out]
  n38 = Unbundle By Name("Config Test IN") -> ("Result"=w5:T5, "Execucion Test.Vasic Actual"=w34:i32)
  n39 = And Array Elements(Boolean array=w8) -> (logical AND=w18:bool)
  n40 = And Array Elements(Boolean array=w9) -> (logical AND=w17:bool)
  n41 = And(x=w17, y=w18) -> (x .and. y?=w16:bool)
  "Min P Max N" <- w16
  n42 = Split Number(x=u16 1855 ("devNum_in")) -> (hi(x)=w41:u8, lo(x)=w40:u8)
  n43 = call "ASIC_WRITE.vi"("ftHandle_in"=w37, "Espera acceso USB"=w35, "Direccion Registro Asic"=u8 101 ("devNum_in"), "Byte Alto"=w41, "Byte Bajo"=w40, "error in"=w36) -> ("ftHandle_out"=w30:u32, "error out"=→"Error OUT":errorcluster)  [unwired: 8 in]
  n44 = Index Array(array=w5, index=w34) -> (element=w33:T6)
  n45 = Bundle By Name(cluster=w33, "Test ADCs.Max P Mini N"=w23, "Test ADCs.Min P Max N"=w16, "Test ADCs.PTHT Max P Min N"=w15, "Test ADCs.Result PTHT Max P Min N"=w11, "Test ADCs.NTHT Max P Min N"=w14, "Test ADCs.Result NTHT Max P Min N"=w10, "Test ADCs.PTHT Max N Min P"=w13, "Test ADCs.Result PTHT Max N Min P"=w9, "Test ADCs.NTHT Max N Min P"=w12, "Test ADCs.Result NTHT Max N Min P"=w8, "Test ADCs.Ref"=w1) -> (w32:T6)
  n46 = Insert Into Array(array=w5, index=w34, new element=w32) -> (w6:T5)
  n47 = Bundle By Name(cluster="Config Test IN", "Result"=w6, "Config HW.FT_Handle"=w30) -> (→"Config Test OUT":T1)
